vi "Run Configuration Script.vi"(8 "error in (no error)":errorcluster, 9 "configuration script":path, 10 "serial channels":string[](array[string]), 11 "fpga interface in":refnum<k20>) -> (0 "error out":errorcluster, 3 "fpga interface out":refnum<k20>)   [LabVIEW 2025, in "I2C Bus Monitor.lvclass"]
uses:
  I2C Bus Monitor.lvclass
  I2C Bus Monitor.lvclass/I2C Bus Monitor.ctl
  <instrlib>/FlexRIO/Automotive Vision Utility/v1/Host/Automotive Vision Utility.lvlib
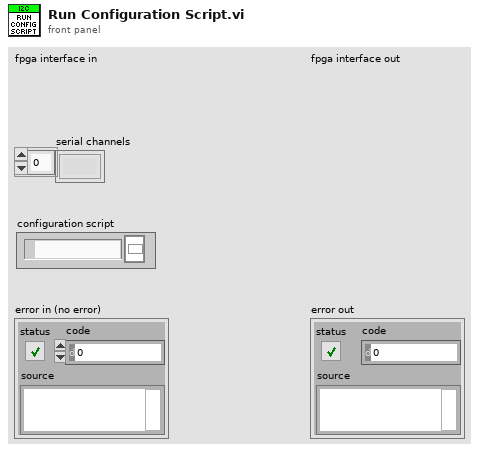
[diagram p1: front panel]
types:
  T1 = typedef "Automotive Vision Utility.lvlib/SerDes Configuration Command.ctl" = cluster{"command type":T2, "address":u16, "write data":u8[], "num bytes to read":u32, "milliseconds to wait":u32}
  T2 = typedef "Automotive Vision Utility.lvlib/SerDes Configuration Command Type.ctl" = enum16{"Wait", "Write", "Transfer", "Read"}
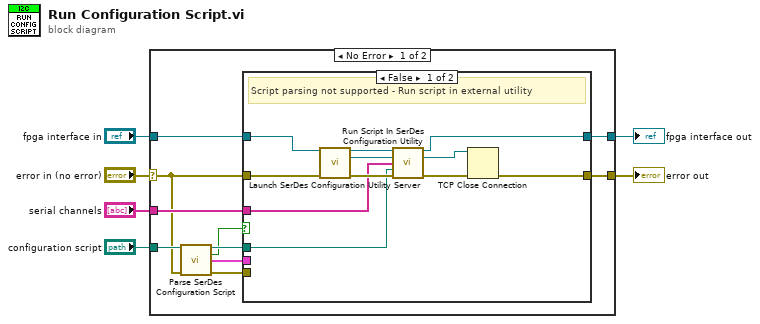
[diagram p0: block diagram]
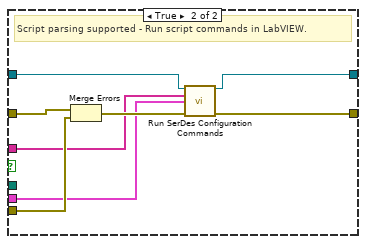
[diagram p2: hidden frame]
diagram:
  n1 = case shown="No Error" "error in (no error)" {
    selector: "error in (no error)" -> [w8 w37]
    tunnel: "fpga interface in" -> [w16 w36]
    tunnel: "serial channels" -> [w15 _]
    tunnel: [w14 w37] -> w4
    tunnel: [w13 w36] -> w3
    tunnel: "configuration script" -> [w12 _]
    frame No Error {
      n2 = call <instrlib>:"Parse SerDes Configuration Script.vi"("configuration script"=w12, "error in"=w8) -> ("configuration script out"=w11:path, "file type supported?"=w7:bool, "serdes config commands"=w10:T1[], "error out"=w9:errorcluster)  [unwired: 10 in]
      n3 = case shown="False" w7 {
        tunnel: w16 -> [w27 w30]
        tunnel: w8 -> [w26 w34]
        tunnel: w15 -> [w22 w28]
        tunnel: w11 -> [w21 _]
        tunnel: [w18 w35] -> w14
        tunnel: [w17 w29] -> w13
        tunnel: w10 -> [_ w31]
        tunnel: w9 -> [_ w32]
        frame False {
          # "Script parsing not supported - Run script in external utility"
          n4 = call <instrlib>:"Launch SerDes Configuration Utility Server.vi"("fpga interface in"=w27, "error in"=w26) -> ("fpga interface out"=w25:refnum<k20>, "socket connection id out"=w24:refnum<k5>, "error out"=w23:errorcluster)  [unwired: 11 in]
          n5 = call <instrlib>:"Run Script In SerDes Configuration Utility.vi"("fpga interface in"=w25, "socket connection id in"=w24, "serial channels"=w22, "configuration script"=w21, "error in"=w23) -> ("fpga interface out"=w17:refnum<k20>, "socket connection id out"=w20:refnum<k5>, "error out"=w19:errorcluster)  [unwired: 8 in]
          n6 = TCP Close Connection(connection ID=w20, error in (no error)=w19) -> (error out=w18:errorcluster)  [unwired: 1 in, 1 out]
        }
        frame True {
          # "Script parsing supported - Run script commands in LabVIEW."
          n7 = Merge Errors(w34, w32) -> (w33:errorcluster)
          n8 = call <instrlib>:"Run SerDes Configuration Commands.vi"("fpga interface in"=w30, "serial channels"=w28, "serdes config commands"=w31, "error in"=w33) -> ("fpga interface out"=w29:refnum<k20>, "error out"=w35:errorcluster)  [unwired: 9 in, 1 out]
        }
      }
    }
    frame Error {
    }
  }
  "fpga interface out" <- w3
  "error out" <- w4
